vi "Load Proto File.vi"(8 "error in (no error)":errorcluster, 10 "Proto File Path":path, 11 "OOP Server in":refnum<class "OOP Server.lvclass">) -> (0 "error out":errorcluster, 3 "OOP Server out":refnum<class "OOP Server.lvclass">)   [LabVIEW 2019, in "OOP Server.lvclass"]
uses:
  OOP Server.lvclass
  typeDefs/Server gRPC UEs.ctl
  gRPC interface/Server API/typeDefs/gRPCId Cluster UE.ctl
  gRPC interface/Server API/typeDefs/gRPCId Cluster.ctl
  gRPC interface/Server API/typeDefs/grpcId.ctl
  gRPC interface/Server API/typeDefs/Message Metadata.ctl
  gRPC interface/Server API/typeDefs/Message Element Metadata.ctl
  gRPC interface/Server API/typeDefs/Message Element Type.ctl
  typeDefs/Server Internal UEs.ctl
  typeDefs/gRPC Server Internal Message.ctl
  OOP Server.lvclass/OOP Server.ctl
  gRPC interface/gprc-lvsupport.lvlib
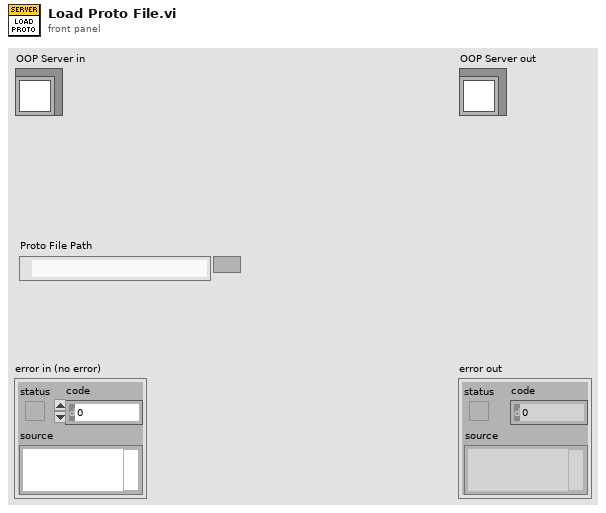
[diagram p1: front panel]
types:
  T1 = typedef "OOP Server.lvclass/Server Internal UEs.ctl" = cluster{"Invoke Internal UE":refnum<user-event>, "Query Internal UE":refnum<user-event>, "Register Internal UE":refnum<user-event>}
  T2 = typedef "gprc-lvsupport.lvlib/Message Metadata.ctl" = cluster{"Name":string, "Elements":T3[]}
  T3 = typedef "gprc-lvsupport.lvlib/Message Element Metadata.ctl" = cluster{"Embedded Message Name":string, "Protobuf Index":i32, "MessageElementType":T4, "Repeated":bool}
  T4 = typedef "gprc-lvsupport.lvlib/Message Element Type.ctl" = enum32{"Int32Value", "FloatValue", "DoubleValue", "BoolValue", "StringValue", "MessageValue", ""}
  T5 = typedef "OOP Server.lvclass/Server gRPC UEs.ctl" = cluster{"Invoke gRPC UEs":T6, "Query gRPC UEs":T6, "Register gRPC UEs":T6}
  T6 = typedef "gprc-lvsupport.lvlib/gRPCId Cluster UE.ctl" = refnum<user-event>
  T7 = typedef "gprc-lvsupport.lvlib/grpcId.ctl" = u64
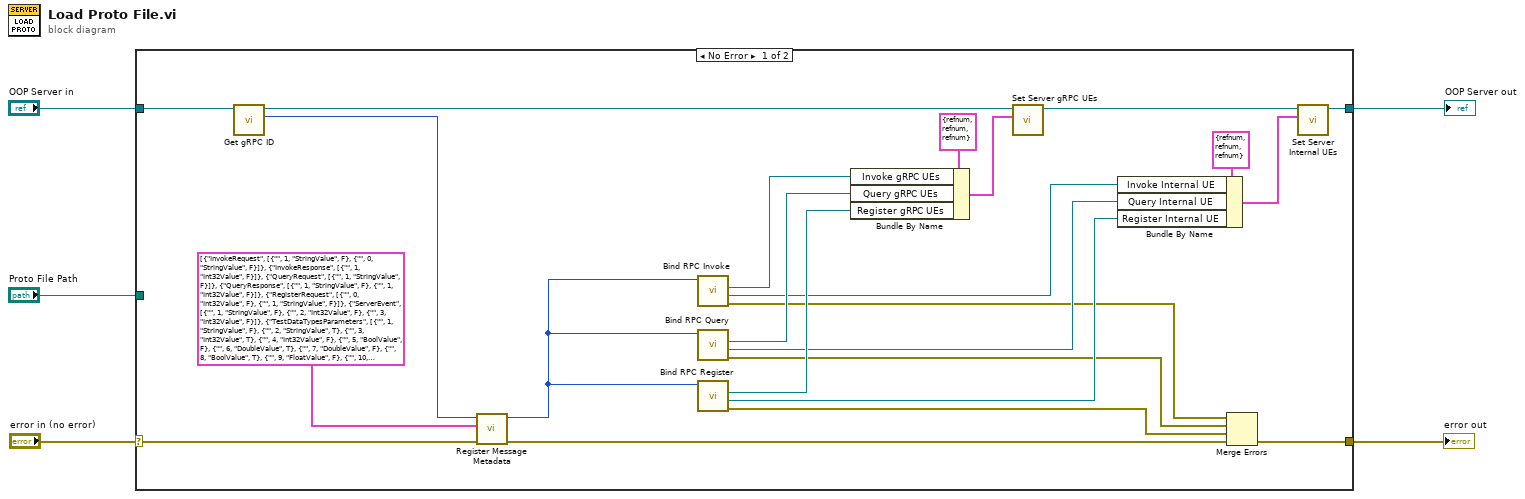
[diagram p0: block diagram]
diagram:
  n1 = case shown="No Error" "error in (no error)" {
    selector: "error in (no error)" -> [w14 w30]
    tunnel: [w6 w30] -> w4
    tunnel: [w16 w29] -> w2
    tunnel: "OOP Server in" -> [w15 w29]
    tunnel: "Proto File Path" -> [_ _]
    frame No Error {
      n2 = call "Get gRPC ID.vi"("OOP Server in"=w15) -> ("gRPC ID"=w12:T7, "OOP Server out"=w13:refnum<class "OOP Server.lvclass">)  [unwired: 9 in]
      n3 = call "Register Message Metadata.vi"("error in (no error)"=w14, "Messages"=T2[] [{"Name"="InvokeRequest", "Elements"=[{"Embedded Message Name"="", "Protobuf Index"=1, "MessageElementType"=enum."StringValue", "Repeated"=FALSE}, {"Embedded Message Name"="", "Protobuf Index"=0, "MessageElementType"=enum."StringValue", "Repeated"=FALSE}]}, {"Name"="InvokeResponse", "Elements"=[{"Embedded Message Name"="", "Protobuf Index"=1, "MessageElementType"=enum."Int32Value", "Repeated"=FALSE}]}, {"Name"="QueryRequest", "Elements"=[{"Embedded Message Name"="", "Protobuf Index"=1, "MessageElementType"=enum."StringValue", "Repeated"=FALSE}]}, {"Name"="QueryResponse", "Elements"=[{"Embedded Message Name"="", "Protobuf Index"=1, "MessageElementType"=enum."StringValue", "Repeated"=FALSE}, {"Embedded Message Name"="", "Protobuf Index"=1, "MessageElementType"=enum."Int32Value", "Repeated"=FALSE}]}, {"Name"="RegisterRequest", "Elements"=[{"Embedded Message Name"="", "Protobuf Index"=0, "MessageElementType"=enum."Int32Value", "Repeated"=FALSE}, {"Embedded Message Name"="", "Protobuf Index"=1, "MessageElementType"=enum."StringValue", "Repeated"=FALSE}]}, {"Name"="ServerEvent", "Elements"=[{"Embedded Message Name"="", "Protobuf Index"=1, "MessageElementType"=enum."StringValue", "Repeated"=FALSE}, {"Embedded Message Name"="", "Protobuf Index"=2, "MessageElementType"=enum."Int32Value", "Repeated"=FALSE}, {"Embedded Message Name"="", "Protobuf Index"=3, "MessageElementType"=enum."Int32Value", "Repeated"=FALSE}]}, {"Name"="TestDataTypesParameters", "Elements"=[{"Embedded Message Name"="", "Protobuf Index"=1, "MessageElementType"=enum."StringValue", "Repeated"=FALSE}, {"Embedded Message Name"="", "Protobuf Index"=2, "MessageElementType"=enum."StringValue", "Repeated"=TRUE}, {"Embedded Message Name"="", "Protobuf Index"=3, "MessageElementType"=enum."Int32Value", "Repeated"=TRUE}, {"Embedded Message Name"="", "Protobuf Index"=4, "MessageElementType"=enum."Int32Value", "Repeated"=FALSE}, {"Embedded Message Name"="", "Protobuf Index"=5, "MessageElementType"=enum."BoolValue", "Repeated"=FALSE}, {"Embedded Message Name"="", "Protobuf Index"=6, "MessageElementType"=enum."DoubleValue", "Repeated"=TRUE}, {"Embedded Message Name"="", "Protobuf Index"=7, "MessageElementType"=enum."DoubleValue", "Repeated"=FALSE}, {"Embedded Message Name"="", "Protobuf Index"=8, "MessageElementType"=enum."BoolValue", "Repeated"=TRUE}, {"Embedded Message Name"="", "Protobuf Index"=9, "MessageElementType"=enum."FloatValue", "Repeated"=FALSE}, {"Embedded Message Name"="", "Protobuf Index"=10, "MessageElementType"=enum."FloatValue", "Repeated"=TRUE}, {"Embedded Message Name"="DataTypeTest", "Protobuf Index"=11, "MessageElementType"=enum."MessageValue", "Repeated"=FALSE}, {"Embedded Message Name"="DataTypeTest", "Protobuf Index"=12, "MessageElementType"=enum."MessageValue", "Repeated"=TRUE}]}, {"Name"="DataTypeTest", "Elements"=[{"Embedded Message Name"="", "Protobuf Index"=1, "MessageElementType"=enum."BoolValue", "Repeated"=FALSE}, {"Embedded Message Name"="", "Protobuf Index"=2, "MessageElementType"=enum."Int32Value", "Repeated"=FALSE}, {"Embedded Message Name"="", "Protobuf Index"=3, "MessageElementType"=enum."FloatValue", "Repeated"=FALSE}, {"Embedded Message Name"="", "Protobuf Index"=4, "MessageElementType"=enum."DoubleValue", "Repeated"=FALSE}]}], "gRPCid"=w12) -> ("error out"=w10:errorcluster, "gRPCid"=w11:T7)  [unwired: 7 in]
      n4 = call "Bind RPC Invoke.vi"("gRPCid server in"=w11) -> ("error out"=w9:errorcluster, "Invoke Internal UE"=w20:refnum<user-event>, "Invoke gRPC UE"=w25:refnum<user-event>)  [unwired: 7 in, 1 out]
      n5 = call "Bind RPC Query.vi"("gRPCid server in"=w11) -> ("error out"=w8:errorcluster, "Query Internal UE"=w19:refnum<user-event>, "Query gRPC UE"=w26:refnum<user-event>)  [unwired: 7 in, 1 out]
      n6 = call "Bind RPC Register.vi"("gRPCid server in"=w11) -> ("error out"=w7:errorcluster, "Register Internal UE"=w18:refnum<user-event>, "Register gRPC UE"=w24:refnum<user-event>)  [unwired: 7 in, 1 out]
      n7 = Bundle By Name(cluster=T5 {"Invoke gRPC UEs"=refnum, "Query gRPC UEs"=refnum, "Register gRPC UEs"=refnum} ("gRPC Server Method Events"), "Invoke gRPC UEs"=w25, "Query gRPC UEs"=w26, "Register gRPC UEs"=w24) -> (w23:T5)
      n8 = call "Set Server gRPC UEs.vi"("Server gRPC UEs"=w23, "OOP Server in"=w13) -> ("OOP Server out"=w22:refnum<class "OOP Server.lvclass">)  [unwired: 9 in]
      n9 = Bundle By Name(cluster=T1 {"Invoke Internal UE"=refnum, "Query Internal UE"=refnum, "Register Internal UE"=refnum} ("Server Internal UEs"), "Invoke Internal UE"=w20, "Query Internal UE"=w19, "Register Internal UE"=w18) -> (w17:T1)
      n10 = Merge Errors(w9, w8, w7, w10) -> (w6:errorcluster)
      n11 = call "Set Server Internal UEs.vi"("Server Internal UEs"=w17, "OOP Server in"=w22) -> ("OOP Server out"=w16:refnum<class "OOP Server.lvclass">)  [unwired: 9 in]
    }
    frame Error {
    }
  }
  "error out" <- w4
  "OOP Server out" <- w2
